vi "IT8800-Query Error.vi"(8 "error in":errorcluster, 11 "IT8800 Setting In In":T1={"VISA Resource Name"="", "Baud Rate"=19200, "Stop Bits"=20, "Wait For Read(ms)"=0} {"Stop Bits" items=["1.0"=10, "2.0"=20]; "Baud Rate" items=["2400"=2400, "4800"=4800, "9600"=9600, "19200"=19200]}) -> (0 "error out":errorcluster, 3 "IT8800 Setting In Out":T1={"VISA Resource Name"="", "Baud Rate"=19200, "Stop Bits"=20, "Wait For Read(ms)"=0} {"Stop Bits" items=["1.0"=10, "2.0"=20]; "Baud Rate" items=["2400"=2400, "4800"=4800, "9600"=9600, "19200"=19200]})   [LabVIEW 2018]
uses:
  Data Def/IT8800-Setting.ctl
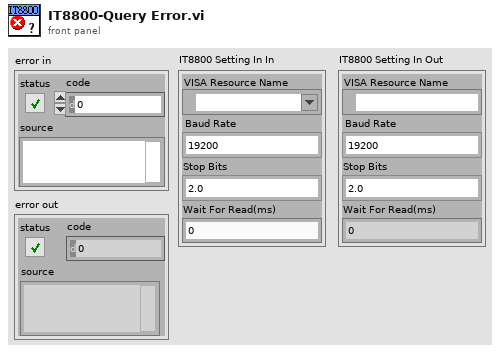
[diagram p1: front panel]
types:
  T1 = typedef "IT8800-Setting.ctl" = cluster{"VISA Resource Name":refnum<visa-resource-name>, "Baud Rate":u32, "Stop Bits":u16, "Wait For Read(ms)":u32}
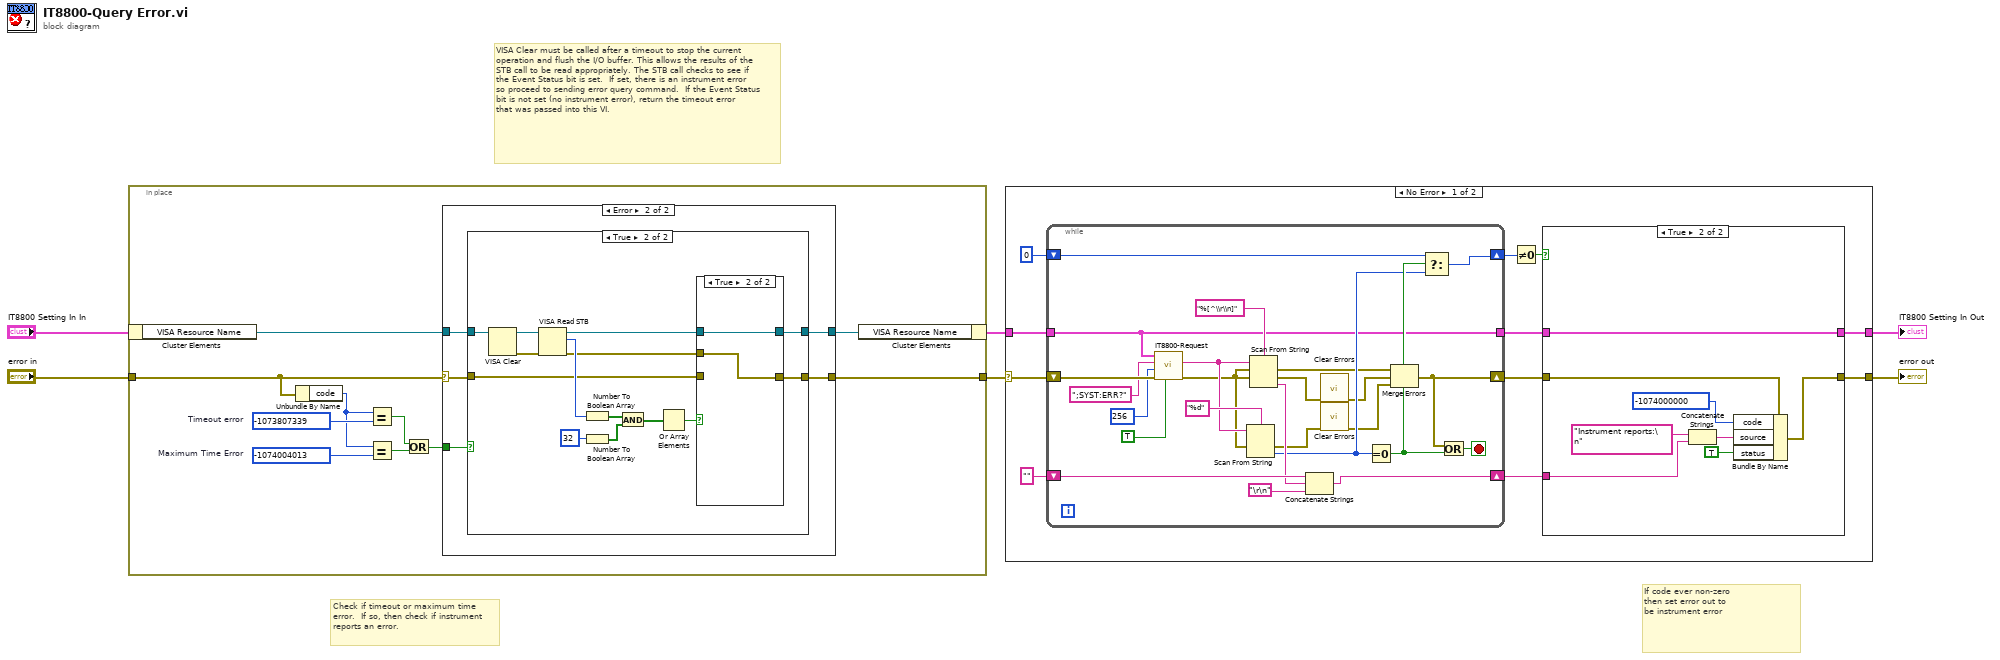
[diagram p0: block diagram]
diagram:
  # "If code ever non-zero\nthen set error out to\nbe instrument error"
  # "Check if timeout or maximum time error.  If so, then check if instrument reports an error."
  # "VISA Clear must be called after a timeout to stop the current operation and flush the I/O buffer. This allows the results of the  STB call to be read appropriately. The STB call checks to see if the Event Status bit is set.  If set, there is an instrument error so proceed to sending error query command.  If the Event Status bit is not set (no instrument error), return the timeout error that was passed into this VI."
  n1 = in-place {
    in-place-border: "error in" -> [w16]
    in-place-border: [w15] -> w4
    w12 = -1074004013  # Maximum Time Error
    w14 = -1073807339  # Timeout error
    n2 = in-place-cluster #1("IT8800 Setting In In") -> ("VISA Resource Name"=w8:refnum<visa-resource-name>)
    n3 = Unbundle By Name(w16) -> ("code"=w13:i32)
    n4 = Equal?(x=w13, y=w14) -> (x = y?=w10:bool)
    n5 = Equal?(x=w13, y=w12) -> (x = y?=w11:bool)
    n6 = Or(x=w10, y=w11) -> (x .or. y?=w9:bool)
    n7 = case shown="Error" w16 {
      selector: w16 -> [w17 w21]
      tunnel: w8 -> [w18 w23]
      tunnel: [w18 w22] -> w7
      tunnel: [w17 w20] -> w15
      tunnel: w9 -> [_ w19]
      frame No Error {
      }
      frame Error {
        n8 = case shown="True" w19 {
          tunnel: w23 -> [w25 w36]
          tunnel: [w25 w26] -> w22
          tunnel: w21 -> [w24 w30]
          tunnel: [w24 w28] -> w20
          frame False {
            # "Error code not a timeout, so best to pass on to user."
          }
          frame True {
            n9 = VISA Clear(VISA resource name=w36) -> (VISA resource name out=w35:refnum<visa-resource-name>, error out=w34:errorcluster)  [unwired: 1 in]
            n10 = VISA Read STB(8:w34, 11:w35) -> (0:w29:errorcluster, 2:w33:u16, 3:w27:refnum<visa-resource-name>)
            n11 = Number To Boolean Array(number=w33) -> (Boolean array=w37:bool[])
            n12 = Number To Boolean Array(number=32) -> (Boolean array=w38:bool[])
            n13 = And(x=w37, y=w38) -> (x .and. y?=w32:bool[])
            n14 = Or Array Elements(Boolean array=w32) -> (logical OR=w31:bool)
            n15 = case shown="True" w31 {
              tunnel: w30 -> [w41 _]
              tunnel: w29 -> [_ w43]
              tunnel: [w41 w43] -> w28
              tunnel: w27 -> [w40 w42]
              tunnel: [w40 w42] -> w26
              frame False {
              }
              frame True {
              }
            }
          }
        }
      }
    }
    n16 = in-place-cluster #1("VISA Resource Name"=w7) -> (w2:T1)
  }
  n17 = case shown="No Error" w4 {
    selector: w4 -> [w48 w88]
    tunnel: [w45 w89] -> w1
    tunnel: w2 -> [w54 w89]
    tunnel: [w44 w88] -> w5
    frame No Error {
      n18 = while {
        tunnel: [w73] -> w46
        tunnel: w54 -> [w73]
        shift-right: [w81] -> w50
        shift-left: "" -> [w84]
        shift-right: [w79] -> w51
        shift-left: 0 -> [w80]
        shift-right: [w76] -> w49
        shift-left: w48 -> [w75]
        stop <- w86 stop-if-true
        n19 = call "IT8800-Request.vi"("Response?"=TRUE, "error in"=w75, "byte count"=u32 256, "Command"=";SYST:ERR?" ("Error Query Command"), "IT8800 Setting In In"=w73) -> ("error out"=w69:errorcluster, "Response"=w72:string)  [unwired: 4 in, 1 out]
        n20 = Scan From String(format string="%d", input string=w72, error in=w69) -> (error out=w67:errorcluster, output 1=w77:i32)  [unwired: 2 in, 2 out]
        n21 = Scan From String(format string="%[^\\r\\n]", input string=w72, error in=w69) -> (error out=w68:errorcluster, output 1=w82:string)  [unwired: 2 in, 2 out]
        n22 = Concatenate Strings(w84, w82, "\r\n") -> (w81:string)
        n23 = call <vilib>:"Clear Errors.vi"("error in (no error)"=w68) -> ("error out"=w66:errorcluster)  [unwired: 5 in, 1 out]
        n24 = call <vilib>:"Clear Errors.vi"("error in (no error)"=w67) -> ("error out"=w65:errorcluster)  [unwired: 5 in, 1 out]
        n25 = Equal To 0?(x=w77) -> (x = 0?=w78:bool)
        n26 = Merge Errors(w69, w66, w65) -> (w76:errorcluster)
        n27 = Select(t=w80, s=w78, f=w77) -> (s? t:f=w79:i32)
        n28 = Or(x=w76, y=w78) -> (x .or. y?=w86:bool)
      }
      n29 = Not Equal To 0?(x=w51) -> (x != 0?=w52:bool)
      n30 = case shown="True" w52 {
        tunnel: w50 -> [_ w63]
        tunnel: [w56 w57] -> w44
        tunnel: w49 -> [w56 w61]
        tunnel: w46 -> [w55 w62]
        tunnel: [w55 w62] -> w45
        frame False {
        }
        frame True {
          n31 = Concatenate Strings("Instrument reports:\n" ("Source"), w63) -> (w60:string)
          n32 = Bundle By Name(cluster=w61, "code"=-1074000000 ("Code"), "source"=w60, "status"=TRUE) -> (w57:errorcluster)
        }
      }
    }
    frame Error {
    }
  }
  "error out" <- w5
  "IT8800 Setting In Out" <- w1
